vi "capture_mode.vi"(8 "error in (no error)":errorcluster, 10 "Capture Mode":string(combo)="Run", 11 "VISA In":refnum<visa-resource-name>) -> (0 "error out":errorcluster, 3 "VISA Out":refnum<visa-resource-name>)   [LabVIEW 2011]
panel:
  out "Selected Mode":string
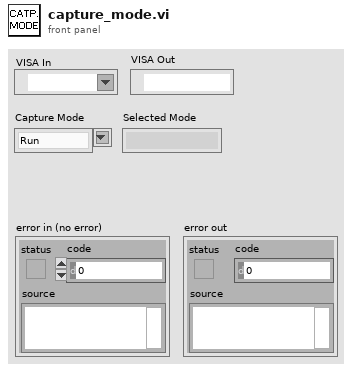
[diagram p1: front panel]
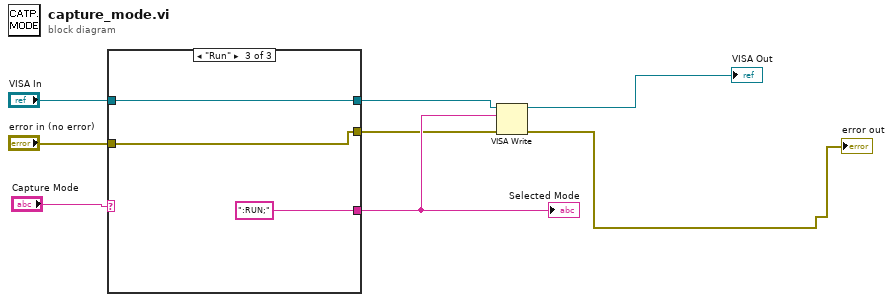
[diagram p0: block diagram]
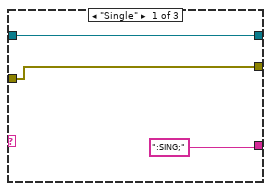
[diagram p2: hidden frame]
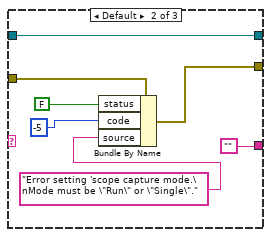
[diagram p3: hidden frame]
diagram:
  n1 = case shown="\"Run\"" "Capture Mode" {
    tunnel: [":SING;" "" ":RUN;"] -> w6
    tunnel: "VISA In" -> [w10 w17 w20]
    tunnel: [w10 w17 w20] -> w4
    tunnel: "error in (no error)" -> [w9 w16 w19]
    tunnel: [w9 w15 w19] -> w2
    frame "Single" {
    }
    frame Default {
      n2 = Bundle By Name(cluster=w16, "status"=FALSE, "code"=-5, "source"="Error setting 'scope capture mode.\nMode must be \"Run\" or \"Single\".") -> (w15:errorcluster)
    }
    frame "Run" {
    }
  }
  "Selected Mode" <- w6
  n3 = VISA Write(VISA resource name=w4, write buffer=w6, error in (no error)=w2) -> (VISA resource name out=→"VISA Out":refnum<visa-resource-name>, error out=→"error out":errorcluster)  [unwired: 1 out]
